vi "read_params.vi"(8 "error in (no error)":errorcluster, 11 "PassiveAggressiveClassifier in":refnum<class "PassiveAggressiveClassifier.lvclass">) -> (0 "error out":errorcluster, 2 "params":T1={"C"=1.0, "fit_intercept"=TRUE, "max_iter"=1000.0, "tol"={"tol_type"="float", "tol_float"=0.001}, "early_stopping"=FALSE, "validation_fraction"=0.1, "n_iter_no_change"=5.0, "shuffle"=TRUE, "verbose"=0.0, "loss"="epsilon_insensitive", "n_jobs"=1.0, "random_state"=0.0, "warm_start"=FALSE, "class_weight"={"class_weight_type"="None", "class_weight_dict"="{1:1.2,2:0.8,3:1.0}"}, "average"=FALSE}, 3 "PassiveAggressiveClassifier out":refnum<class "PassiveAggressiveClassifier.lvclass">)   [LabVIEW 2020, in "PassiveAggressiveClassifier.lvclass"]
uses:
  PassiveAggressiveClassifier.lvclass
  Controls/passive_aggressive_classifier_params.ctl
  PassiveAggressiveClassifier.lvclass/PassiveAggressiveClassifier.ctl
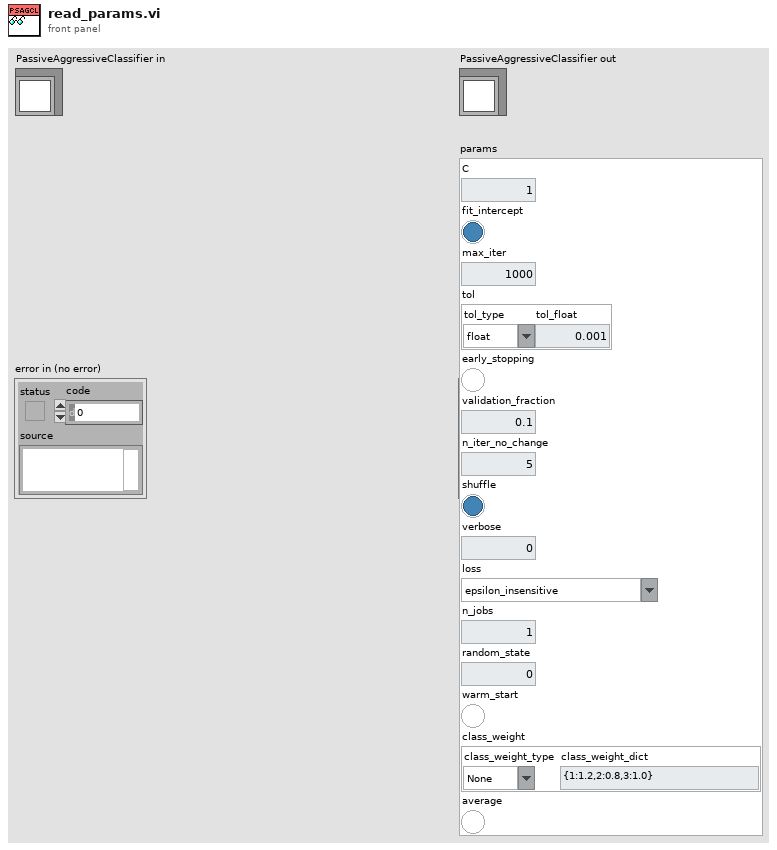
[diagram p1: front panel]
types:
  T1 = typedef "passive_aggressive_classifier_params.ctl" = cluster{"C":dbl, "fit_intercept":bool, "max_iter":dbl, "tol":cluster{"tol_type":string, "tol_float":dbl}, "early_stopping":bool, "validation_fraction":dbl, "n_iter_no_change":dbl, "shuffle":bool, "verbose":dbl, "loss":string, "n_jobs":dbl, "random_state":dbl, "warm_start":bool, "class_weight":cluster{"class_weight_type":string, "class_weight_dict":string}, "average":bool}
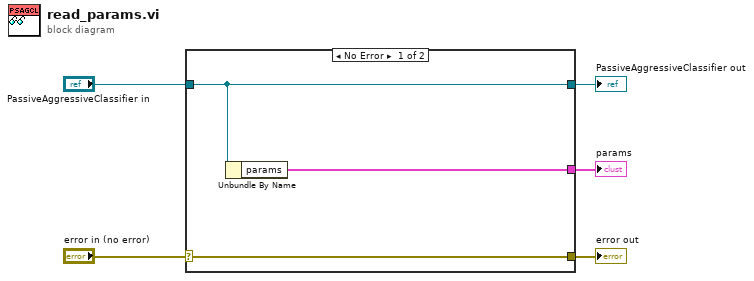
[diagram p0: block diagram]
diagram:
  n1 = case shown="No Error" "error in (no error)" {
    selector: "error in (no error)" -> [w8 w9]
    tunnel: [w8 w9] -> w4
    tunnel: [w7 w10] -> w2
    tunnel: "PassiveAggressiveClassifier in" -> [w7 w10]
    tunnel: [w6 _] -> w1
    frame No Error {
      n2 = Unbundle By Name(w7) -> ("params"=w6:T1)
    }
    frame Error {
    }
  }
  "error out" <- w4
  "PassiveAggressiveClassifier out" <- w2
  "params" <- w1
